vi "Globales Snake.vi"() -> ()   [LabVIEW 2021]
panel:
  in  "player name":string
  out "Game Running":bool
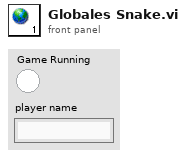
[diagram p1: front panel]
diagram:
